vi "NaOvenTempToInflux.vi"(3 "error in (no error)":errorcluster, 4 "Temperature Input":dbl, 5 "Thermocouple":u16(ring) items=["Sodium Cup (T1)", "Flange (T2)"]) -> (0 "error out":errorcluster, 1 "InfluxDB Comm Error":bool)   [LabVIEW 2013, in "ovenCtrl.lvlib"]
uses:
  ovenCtrl.lvlib
panel:
  out "Reading Time":timestamp
  # "Inputs"
  # "Outputs"
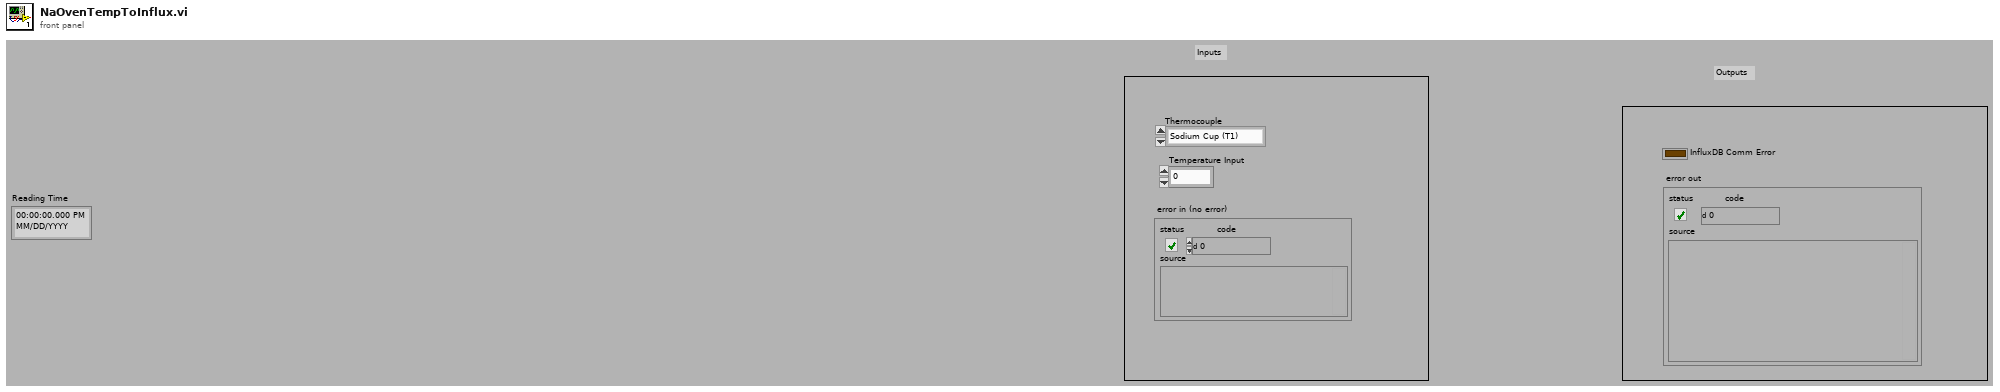
[diagram p1: front panel]
types:
  T1 = cluster{"ReadingTimestamp":timestamp, "Numeric Input":dbl}
  T2 = cluster{"DBWrite":string, "Auth":string, "EventsBody":string, "CurrentBody":string}
  T3 = cluster{"InfluxDB Address":string, "InfluxDB Database":string, "InfluxDB Base64 Credentials":string}
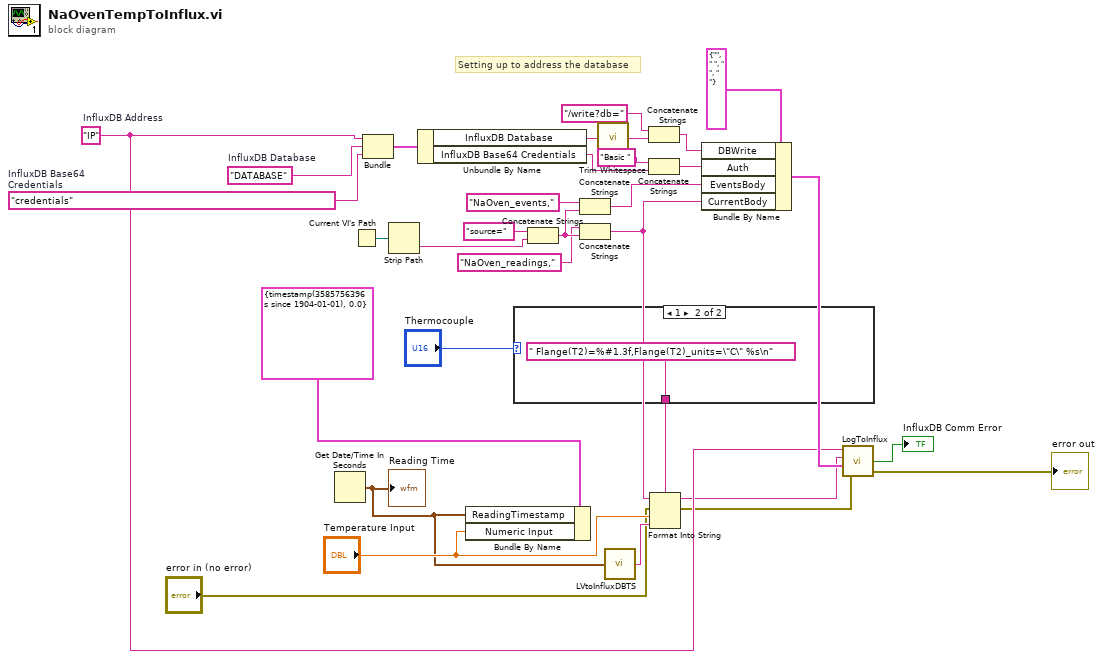
[diagram p0: block diagram]
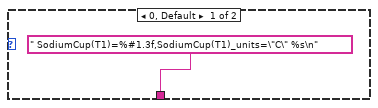
[diagram p2: hidden frame]
diagram:
  w31 = "credentials"  # InfluxDB Base64 Credentials
  w32 = "DATABASE"  # InfluxDB Database
  w6 = "IP"  # InfluxDB Address
  # "Setting up to address the database"
  n1 = Get Date/Time In Seconds() -> (seconds since 1Jan1904=w12:timestamp)
  "Reading Time" <- w12
  n2 = Current VI's Path() -> (path=w22:path)
  n3 = Bundle("InfluxDB Address"=w6, "InfluxDB Database"=w32, "InfluxDB Base64 Credentials"=w31) -> (w15:T3)  [unwired: 1 in]
  n4 = Strip Path(path=w22) -> (name=w20:string)  [unwired: 1 out]
  n5 = Unbundle By Name(w15) -> ("InfluxDB Database"=w28:string, "InfluxDB Base64 Credentials"=w30:string)
  n6 = Bundle By Name(cluster=T1 {"ReadingTimestamp"=timestamp(3585756396.2608747 s since 1904-01-01), "Numeric Input"=0.0}, "ReadingTimestamp"=w12, "Numeric Input"="Temperature Input") -> ()  [unwired: 1 out]
  n7 = case shown="1" "Thermocouple" {
    tunnel: [" SodiumCup(T1)=%#1.3f,SodiumCup(T1)_units=\"C\" %s\n" " Flange(T2)=%#1.3f,Flange(T2)_units=\"C\" %s\n"] -> w9
    frame 0, Default {
    }
    frame 1 {
    }
  }
  n8 = Concatenate Strings("source=" ("string"), w20) -> (w19:string)
  n9 = Concatenate Strings("NaOven_events," ("string"), w19) -> (w18:string)
  n10 = Concatenate Strings("NaOven_readings," ("string"), w19) -> (w8:string)
  n11 = call <vilib>:"Trim Whitespace.vi"("string"=w28) -> ("trimmed string"=w27:string)  [unwired: 1 in]
  n12 = call "LVtoInfluxDBTS.vi"("LV Timestamp"=w12) -> ("InfluxDB ns Timestamp"=w11:string)
  n13 = Concatenate Strings("/write?db=" ("format string"), w27) -> (w25:string)
  n14 = Concatenate Strings("Basic " ("string"), w30) -> (w24:string)
  n15 = Format Into String(format string=w9, initial string=w8, error in="error in (no error)", "Temperature Input", w11) -> (resulting string=w5:string, error out=w2:errorcluster)
  n16 = Bundle By Name(cluster=T2 {"DBWrite"="", "Auth"=" ", "EventsBody"=" ", "CurrentBody"=" "} ("input cluster"), "DBWrite"=w25, "Auth"=w24, "EventsBody"=w18, "CurrentBody"=w8) -> (w7:T2)
  n17 = call "LogToInflux.vi"("error in (no error)"=w2, "InfluxDB Info"=w7, "InfluxDB Line Protocol"=w5, "InfluxDB Address"=w6) -> ("error out"=→"error out":errorcluster, "InfluxDB"=→"InfluxDB Comm Error":bool)  [unwired: 1 out]
